vi "PostStop - Triaxial Shear (SubVI).vi"(8 "error in (no error)":errorcluster, 11 "Cluster in in":T1 {"M Event" items=["Stop", "Running", "PID", "Up Limit", "Down Limit", "Load Limit"]; "Test Type" items=["Please Select", "Triaxial Shear", "Triaxial UU", "Shearbox", "Permeability", "Consolidation (Stepped Loading)/Swelling", "Saturation (Incremental)", "User Defined", "UCT", "Isotropic Consolidation", "Swelling Pressure"]; "Data"."Test Type" items=["Please Select", "Triaxial Shear", "Triaxial UU", "Shearbox", "Permeability", "Consolidation (Stepped Loading)/Swelling", "Saturation (Incremental)", "User Defined", "UCT", "Isotropic Consolidation", "Swelling Pressure"]}) -> (0 "error out":errorcluster, 2 "Enum":T10, 3 "Cluster out":T1 {"M Event" items=["Stop", "Running", "PID", "Up Limit", "Down Limit", "Load Limit"]; "Test Type" items=["Please Select", "Triaxial Shear", "Triaxial UU", "Shearbox", "Permeability", "Consolidation (Stepped Loading)/Swelling", "Saturation (Incremental)", "User Defined", "UCT", "Isotropic Consolidation", "Swelling Pressure"]; "Data"."Test Type" items=["Please Select", "Triaxial Shear", "Triaxial UU", "Shearbox", "Permeability", "Consolidation (Stepped Loading)/Swelling", "Saturation (Incremental)", "User Defined", "UCT", "Isotropic Consolidation", "Swelling Pressure"]})   [LabVIEW 2019]
uses:
  Controls/RunTest - State.ctl
  Controls/RunTest - Data Structure.ctl
  Controls/Test Panel - Data Structure.ctl
  Controls/Station - Test Type.ctl
  <vilib>/Utility/miscctls.llb/LVRowAndColumnTypeDef.ctl
  Controls/RunTest - Calculate Data.ctl
  <vilib>/httpClient/ClientHandle.ctl
  Controls/RunTest - Start Condition.ctl
  Controls/RunTest - Stop Condition.ctl
  Controls/UDP - Event.ctl
  Controls/UDP - Command.ctl
  <vilib>/httpClient/LabVIEWHTTPClient.lvlib
panel:
  out "BP LastValue":sgl
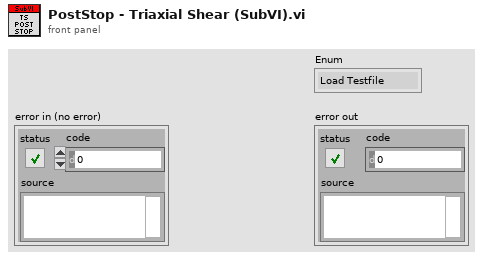
[diagram p1: front panel]
types:
  T1 = typedef "RunTest - Data Structure.ctl" = cluster{"Test Plan":string[], "PlanRow":i32, "Device Name":string[], "Timeout":i32, "Start?":bool, "Pause?":bool, "IP Address":string[], "LogRow":i32, "Logtype":u16, "Log Elapse":sgl, "Data":T2, "Stop log?":bool, "tdms":refnum<k34>, "Sensor Data":sgl[], "Start time":timestamp, "Prev Log Elapse":u32, "Plot":u16, "X-Axis":u16[], "Y-Axis":u16[], "XY":cluster{"X":dbl, "Y":dbl}[][], "End Stage?":bool, "1run":bool, "Condition":u16[], "Start Con":bool, "Log Con":bool, "Stop Con":bool, "Start Elapse":dbl, "Start Load":dbl, "Motor":i32, "StartRow":i32, "number log":i32, "Dir":bool, "Start time test":timestamp, "Auto":bool, "Check return?":bool, "Inv":cluster{"M":i32[], "Bool":bool[]}, "tdms temp":refnum<k34>, "Zero?":bool, "Plot Timer":dbl, "1st Run":bool, "TDMS Path":path, "MaxLoad":dbl, "Log Timer":sgl[], "Test Type":T3, "Log Sensor":string[], "Save?":bool, "1st Log":bool, "Y-Axis 2":u16[], "On Y-Axis 2":bool, "Decimal":u8[], "Init":cluster{"PWP TS":sgl, "Load TS":sgl, "Volume TS":sgl, "Disp TS":sgl, "CP":sgl, "Vol In":sgl, "Vol Out":sgl, "Load UCT":sgl, "Disp UCT":sgl, "PWP Sat":sgl, "CP Sat":sgl, "Volume IsoCons":sgl, "PWP IsoCons":sgl, "PWP TUU":sgl, "Load TUU":sgl, "Volume TUU":sgl, "Disp TUU":sgl, "Load Cons":sgl, "Disp Cons":sgl, "Volume Sat":sgl, "Vertical Load SB":sgl, "Vertical Disp SB":sgl, "H Disp SB":sgl, "H Load SB":sgl}, "Calc":T5, "Device Index":i32[], "Channel Index":i32[], "http ref":T6, "fileid":string, "Step Cons":cluster{"V Stress":sgl, "H Settlement":sgl}, "RunTest":bool, "Graph Last":i32, "Init?":bool, "Datalog":bool[], "Start":T7, "Stop":T8, "Running?":bool, "StartTime":dbl, "Log Prev Time":dbl, "KeyName":string[], "Test RunTime":dbl, "Log Prev Axial":dbl, "M Event":T9[], "Last Log":bool, "popup":bool, "PreStart UU":bool, "PreStart Sat":bool}
  T2 = typedef "Test Panel - Data Structure.ctl" = cluster{"Station":string, "Sample ID":string, "Job No":string, "Job Description":string, "Filename":string, "Test Type":T3, "Speciment No":string, "Depth":string, "Height":string, "Diameter/Length":string, "Weight":string, "Test Parameter":string, "Station[]":string[], "Edit Pos":T4, "Edit Pos Prev":T4, "Area":string, "Path":string}
  T3 = typedef "Station - Test Type.ctl" = u16
  T4 = typedef "LVRowAndColumnTypeDef.ctl" = cluster{"Row":i32, "Column":i32}
  T5 = typedef "RunTest - Calculate Data.ctl" = cluster{"TS":cluster{"Change PWP":sgl, "Change Vol":sgl, "Axial Load":sgl, "CiL":sgl, "Deviator":sgl, "Axial Strain":sgl, "MaxDeviator":sgl}, "TUU":cluster{"Change PWP":sgl, "Axial Load":sgl, "CiL":sgl, "Deviator":sgl, "Axial Strain":sgl, "MaxDeviator":sgl}, "Sat":cluster{"B Value":sgl, "PWP Diss":sgl, "CPP":sgl, "CV":sgl}, "Per":cluster{"Change Vol In":sgl, "Change Vol Out":sgl, "Mean Vol":sgl, "Gradient Pressure":sgl, "Outlet Flow":sgl, "Inlet Flow":sgl, "I X1":sgl, "I X2":sgl, "I Y1":sgl, "I Y2":sgl, "O X1":sgl, "O X2":sgl, "O Y1":sgl, "O Y2":sgl}, "Step Cons":cluster{"V Stress":sgl, "H Settlement":sgl, "Total H Settle":sgl, "Prev Total H":sgl}, "UCT":cluster{"ALC":sgl, "H Change":sgl, "Deviator":sgl, "Axial Strain":sgl, "V Stress":sgl, "MaxDeviator":sgl}, "ISO Cons":cluster{"CPP":sgl, "PWP Diss":sgl, "CV":sgl}, "SB":cluster{"Speci LenC":sgl, "Shear Strain":sgl, "H LC":sgl, "Normal Stress":sgl, "Shear Stress":sgl, "MaxShear":sgl}}
  T6 = typedef "LabVIEWHTTPClient.lvlib/ClientHandle.ctl" = refnum<k1>
  T7 = typedef "RunTest - Start Condition.ctl" = cluster{"Cons":cluster{"VS":dbl, "Delay":bool, "No Delay":dbl}, "Sat":cluster{"CP":dbl, "BP":dbl, "StartBP":bool, "Target CP":bool, "Target BP":bool}, "Iso":cluster{"Select":dbl, "BP":dbl, "IC2":dbl, "IC3":dbl, "IC4":dbl, ". IC6":bool, "IC6":dbl, "IC6-2":dbl, "Target":bool, "Time Cond":dbl, "Last PWP":dbl}, "TS":cluster{"SS":dbl, "Engage":bool, "ES":dbl, "LC":dbl, "PreStart":bool, "Trig SS":bool, "Drain":dbl}, "TUU":cluster{"SS":dbl, "Engage":bool, "ES":dbl, "LC":dbl, "PreStart":bool, "Trig SS":bool, "CP":dbl, "Delay Value":dbl, "Delay":bool, "CP PID":bool}, "UCT":cluster{"SS":dbl, "Engage":bool, "ES":dbl, "LC":dbl, "PreStart":bool, "Trig SS":bool}, "Enable?":bool, "SB":cluster{"SS":dbl, "Engage":bool, "ES":dbl, "LC":dbl, "PreStart":bool, "Trig SS":bool, "VS":dbl, "Delay Value":dbl, "Delay":bool, "VS PID":bool}, "Perm":cluster{"DP":dbl}}
  T8 = typedef "RunTest - Stop Condition.ctl" = cluster{"Cons":cluster{"Select":i32, "Disp":dbl, "Time":dbl, "Time2":dbl, "Disp 2":dbl, "Time Cond":dbl, "Last Disp":dbl, "Swell":bool}, "Sat":cluster{"Select":i32, "PP":dbl, "Time":dbl, "VC":dbl, "Time2":dbl, "Time Cond":dbl, "Last PP":dbl, ".B":bool, "B":dbl, "Last Vc":dbl, "Time Cond 2":dbl, "Time3":dbl, "Time Cond 3":dbl, "B Achieve":bool}, "Iso":cluster{"PP":dbl, "Time":dbl, "VC":dbl, "Time2":dbl, "Time Cond":dbl, "Last Vc":dbl, ".PP":bool, "Time Cond 2":dbl, "Select":i32}, "TS":cluster{"Axial":dbl, ".MaxDev":bool, "MaxDev Value":dbl, "Return":bool, "Reset":bool, "Prev Time":dbl, "PostStop Run":bool, "CP Stop":bool, "BP Stop":bool, "PostStop Trig":bool, "Reset Value":dbl, "BPTrig":bool, "CPTrig":bool, "VLCTrig":bool}, "TUU":cluster{"Axial":dbl, ".MaxDev":bool, "MaxDev Value":dbl, "Return":bool, "Reset":bool, "Prev Time":dbl, "PostStop Run":bool, "CP Stop":bool, "BP Stop":bool, "PostStop Trig":bool, "Reset Value":dbl, "BPTrig":bool, "CPTrig":bool, "VLCTrig":bool}, "UCT":cluster{"Axial":dbl, ".MaxDev":bool, "MaxDev Value":dbl, "Return":bool, "Reset":bool, "Prev Time":dbl, "PostStop Run":bool, "CP Stop":bool, "BP Stop":bool, "PostStop Trig":bool}, "Enable?":bool, "SB":cluster{"Shear":dbl, ".MaxShear":bool, "MaxShear Value":dbl, "Return":bool, "Reset":bool, "Prev Time":dbl, "PostStop Run":bool, "CP Stop":bool, "BP Stop":bool, "PostStop Trig":bool, "Reset Value":dbl, "BPTrig":bool, "CPTrig":bool, "VLCTrig":bool}, "Perm":cluster{"Max Time":bool, "Reset":bool, "PostStop Run":bool, "Ratio":bool, "Reset Value":dbl, "Time":dbl, "RatioTime":dbl, "RatioMore":dbl, "RatioLess":dbl, "Time Cond":dbl, "Time Cond 2":dbl, "Prev IF":dbl, "Prev OF":dbl, "PostStop Trig":bool, "BP Trig":bool, "DP Stop":bool, "BP Stop":bool, "CP Stop":bool, "CP Trig":bool}, "SP":cluster{".Max Time":bool, ".Time":bool, "Time":dbl, "MaxTime":dbl, "Time Cond":dbl, "Max Time Cond":dbl, "Stress":dbl}}
  T9 = typedef "UDP - Event.ctl" = u16
  T10 = typedef "RunTest - State.ctl" = enum16{"Load Testfile", "Notifier", "Init", "Idle", "Load", "Read DB", "Run", "Pause", "Stop", "Check Start", "Check Stop", "Check Post Stop", "Check Log", "EndStage", "Data View", "Display", "Graph", "Graph Old", "Close", "Stop PID", "Check Limit", "Auto", "Up", "Log", "Zero", "Machine Control", "Save Report"}
  T11 = typedef "UDP - Command.ctl" = enum16{"Stop", "Jog Up", "Jog Down", "Ramp Up", "Ramp Down", "PID Target", "PID Ramp", "Disp Run", "Read Ch Data", "Zero Channel", "Zero Disp", "Read Sensor", "Write Sensor", "Read ADC", "Write ADC", "Read PID", "Write PID", "Read Test", "Write Test", "Read System", "Write System", "Read Datalog", "Read Datalog Sensor"}
  T12 = cluster{"Target Load":sgl, "Target Disp":sgl, "Rate":sgl, "Speed":sgl}
  T13 = enum16{"None", "Run Target", "Run Ramp", "Run Disp"}
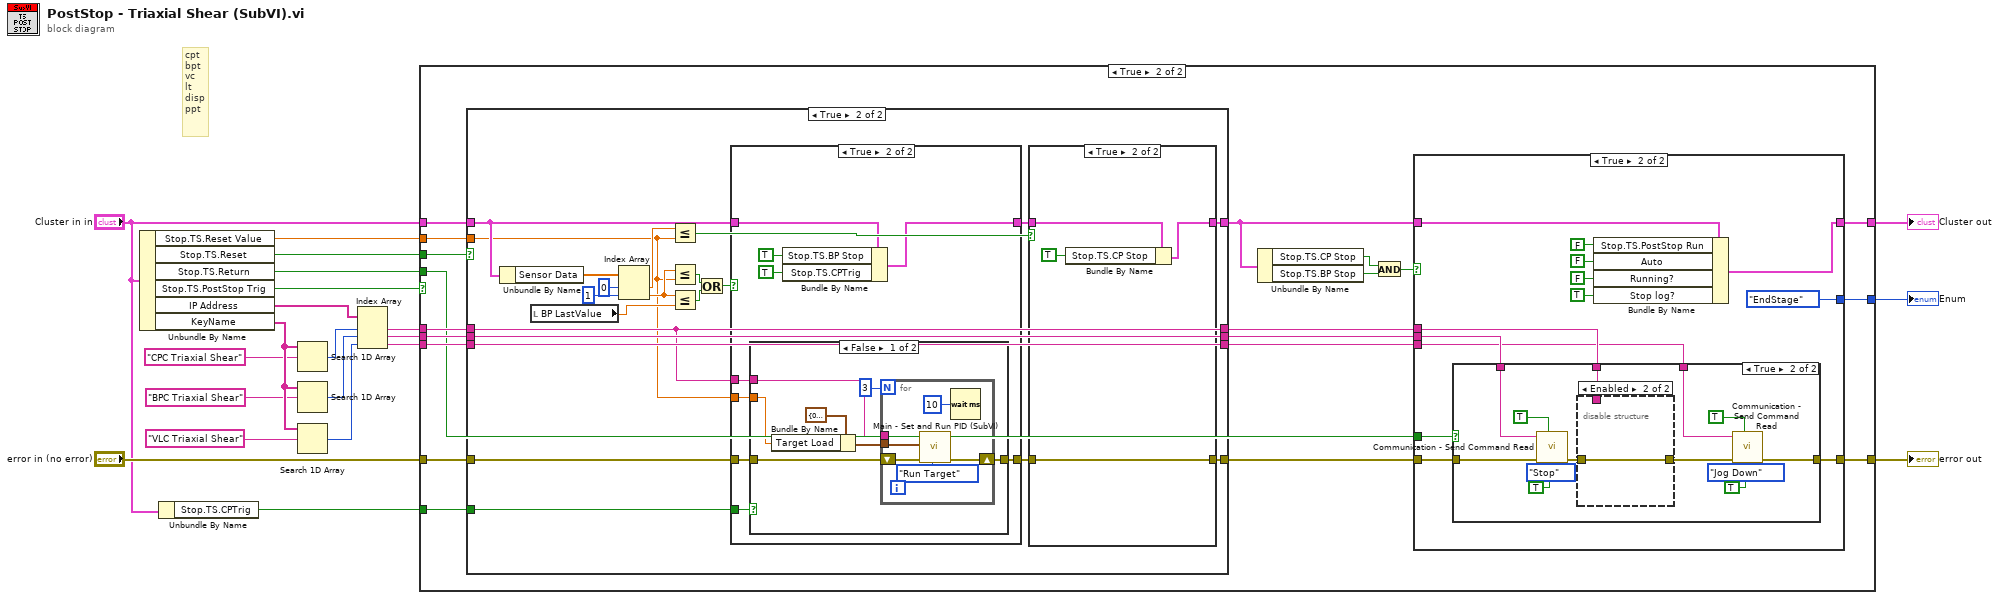
[diagram p0: block diagram]
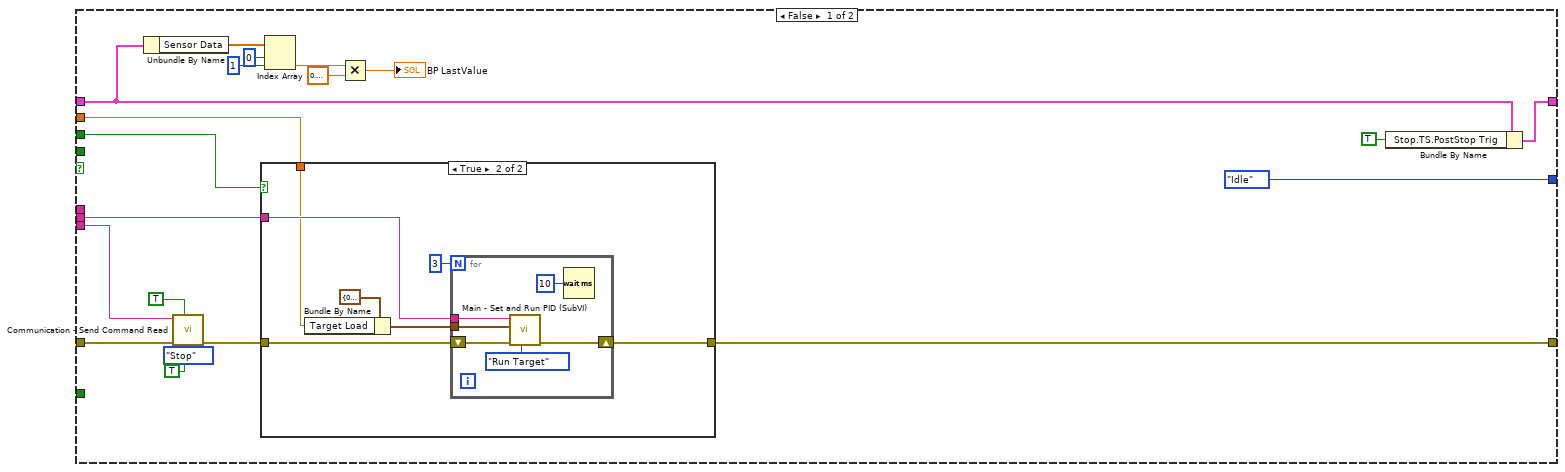
[diagram p2: hidden frame]
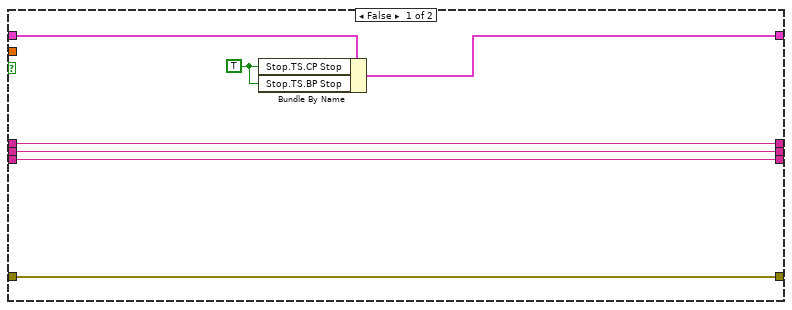
[diagram p4: hidden frame]
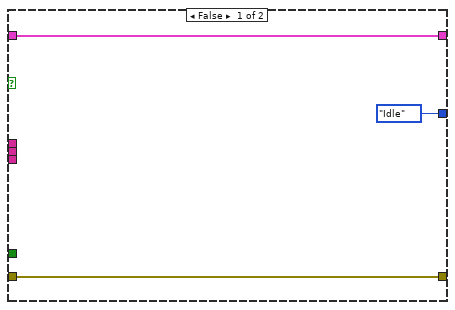
[diagram p8: hidden frame]
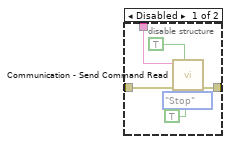
[diagram p10: hidden frame]
diagram:
  # "cpt\nbpt\nvc\nlt\ndisp\nppt"
  n1 = Unbundle By Name("Cluster in in") -> ("Stop.TS.Reset Value"=w21:dbl, "Stop.TS.Reset"=w19:bool, "Stop.TS.Return"=w18:bool, "Stop.TS.PostStop Trig"=w3:bool, "IP Address"=w20:string[], "KeyName"=w16:string[])
  n2 = Unbundle By Name("Cluster in in") -> ("Stop.TS.CPTrig"=w1:bool)
  n3 = Search 1D Array(1D array=w16, element="CPC Triaxial Shear" ("String")) -> (index of element=w9:i32)  [unwired: 1 in]
  n4 = Search 1D Array(1D array=w16, element="BPC Triaxial Shear" ("String")) -> (index of element=w10:i32)  [unwired: 1 in]
  n5 = Search 1D Array(1D array=w16, element="VLC Triaxial Shear" ("String")) -> (index of element=w15:i32)  [unwired: 1 in]
  n6 = Index Array(array=w20, index #1=w9, index #2=w10, index #3=w15) -> (element #1=w11:string, element #2=w12:string, element #3=w17:string)
  n7 = case shown="True" w3 {
    tunnel: [w41 w69] -> w4
    tunnel: "Cluster in in" -> [w25 w71]
    tunnel: [w32 w67] -> w6
    tunnel: "error in (no error)" -> [w35 w75]
    tunnel: w11 -> [_ w74]
    tunnel: w12 -> [w31 w73]
    tunnel: [RunTest_-_State."Idle" w72] -> w13
    tunnel: w17 -> [w34 w59]
    tunnel: w18 -> [_ w57]
    tunnel: w19 -> [w39 w56]
    tunnel: w21 -> [w30 w63]
    tunnel: w1 -> [_ w62]
    frame False {
      n8 = Unbundle By Name(w25) -> ("Sensor Data"=w28:sgl[])
      n9 = call "Communication - Send Command Read.vi"("Fron?"=TRUE, "Bypass?"=TRUE, "error in (no error)"=w35, "Action"=UDP_-_Command."Stop", "Device IP Address"=w34) -> ("error out"=w33:errorcluster)  [unwired: 6 in]
      n10 = case shown="True" w39 {
        tunnel: w33 -> [w42 w47]
        tunnel: w31 -> [_ w46]
        tunnel: [w42 w44] -> w32
        tunnel: w30 -> [_ w45]
        frame False {
        }
        frame True {
          n11 = Bundle By Name(cluster=T12 {"Target Load"=0.0, "Target Disp"=0.0, "Rate"=0.0, "Speed"=0.0} ("Test"), "Target Load"=w45) -> (w48:T12)
          n12 = for {
            N: 3 -> [_]
            tunnel: w48 -> [w54]
            tunnel: w46 -> [w52]
            shift-right: [w51] -> w44
            shift-left: w47 -> [w53]
            n13 = call "Main - Set and Run PID (SubVI).vi"("Action"=T13."Run Target", "error in (no error)"=w53, "Test"=w54, "IP Address"=w52) -> ("error out"=w51:errorcluster)  [unwired: 7 in]
            n14 = Wait (ms)(milliseconds to wait=u32 10) -> ()  [unwired: 1 out]
          }
        }
      }
      n15 = Index Array(array=w28, index #1=0 ("index"), index #2=1 ("index")) -> (element #2=w24:sgl)  [unwired: 1 out]
      n16 = Multiply(x=w24, y=sgl 0.3) -> (x*y=→"BP LastValue":sgl)
      n17 = Bundle By Name(cluster=w25, "Stop.TS.PostStop Trig"=TRUE) -> (w41:T1)
    }
    frame True {
      n18 = case shown="True" w56 {
        tunnel: w75 -> [w79 w103]
        tunnel: w74 -> [w78 w89]
        tunnel: w73 -> [w77 w91]
        tunnel: w71 -> [w81 w102]
        tunnel: [w80 w101] -> w68
        tunnel: [w79 w100] -> w66
        tunnel: w63 -> [_ w86]
        tunnel: w62 -> [_ w92]
        tunnel: [w78 w89] -> w61
        tunnel: [w77 w91] -> w60
        tunnel: w59 -> [w76 w90]
        tunnel: [w76 w90] -> w58
        frame False {
          w82 = TRUE ("Stop.TS.CP Stop")
          n19 = Bundle By Name(cluster=w81, "Stop.TS.CP Stop"=w82, "Stop.TS.BP Stop"=w82) -> (w80:T1)
        }
        frame True {
          n20 = Unbundle By Name(w102) -> ("Sensor Data"=w99:sgl[])
          n21 = local read "BP LastValue"() -> (w88:sgl)
          n22 = Index Array(array=w99, index #1=0 ("index"), index #2=1 ("index")) -> (element #1=w94:sgl, element #2=w87:sgl)
          n23 = Less Or Equal?(x=w94, y=w86) -> (x <= y?=w93:bool)
          n24 = Less Or Equal?(x=w87, y=w86) -> (x <= y?=w85:bool)
          n25 = Less Or Equal?(x=w87, y=w88) -> (x <= y?=w84:bool)
          n26 = Or(x=w85, y=w84) -> (x .or. y?=w83:bool)
          n27 = case shown="True" w83 {
            tunnel: w103 -> [w111 w113]
            tunnel: [w111 w117] -> w96
            tunnel: w102 -> [w110 w120]
            tunnel: [w110 w118] -> w95
            tunnel: w89 -> [_ w116]
            tunnel: w86 -> [_ w115]
            tunnel: w92 -> [_ w114]
            frame False {
            }
            frame True {
              n28 = case shown="False" w114 {
                tunnel: w113 -> [w125 w134]
                tunnel: [w124 w134] -> w117
                tunnel: w116 -> [w123 _]
                tunnel: w115 -> [w122 _]
                frame False {
                  n29 = Bundle By Name(cluster=T12 {"Target Load"=0.0, "Target Disp"=0.0, "Rate"=0.0, "Speed"=0.0} ("Test"), "Target Load"=w122) -> (w127:T12)
                  n30 = for {
                    N: 3 -> [_]
                    tunnel: w127 -> [w133]
                    tunnel: w123 -> [w129]
                    shift-right: [w130] -> w124
                    shift-left: w125 -> [w131]
                    n31 = call "Main - Set and Run PID (SubVI).vi"("Action"=T13."Run Target", "error in (no error)"=w131, "Test"=w133, "IP Address"=w129) -> ("error out"=w130:errorcluster)  [unwired: 7 in]
                    n32 = Wait (ms)(milliseconds to wait=u32 10) -> ()  [unwired: 1 out]
                  }
                }
                frame True {
                }
              }
              n33 = Bundle By Name(cluster=w120, "Stop.TS.BP Stop"=TRUE, "Stop.TS.CPTrig"=TRUE) -> (w118:T1)
            }
          }
          n34 = case shown="True" w93 {
            tunnel: w96 -> [w105 w106]
            tunnel: [w105 w106] -> w100
            tunnel: w95 -> [w104 w108]
            tunnel: [w104 w107] -> w101
            frame False {
            }
            frame True {
              n35 = Bundle By Name(cluster=w108, "Stop.TS.CP Stop"=TRUE ("Stop.TS.BP Stop")) -> (w107:T1)
            }
          }
        }
      }
      n36 = Unbundle By Name(w68) -> ("Stop.TS.CP Stop"=w65:bool, "Stop.TS.BP Stop"=w64:bool)
      n37 = And(x=w65, y=w64) -> (x .and. y?=w70:bool)
      n38 = case shown="True" w70 {
        tunnel: [RunTest_-_State."Idle" RunTest_-_State."EndStage"] -> w72
        tunnel: [w136 w147] -> w69
        tunnel: w68 -> [w136 w149]
        tunnel: [w135 w141] -> w67
        tunnel: w66 -> [w135 w144]
        tunnel: w61 -> [_ w143]
        tunnel: w60 -> [_ w142]
        tunnel: w58 -> [_ w140]
        tunnel: w57 -> [_ w139]
        frame False {
        }
        frame True {
          n39 = case shown="True" w139 {
            tunnel: w144 -> [w151 w160]
            tunnel: w143 -> [_ w159]
            tunnel: w142 -> [_ w158]
            tunnel: [w151 w153] -> w141
            tunnel: w140 -> [_ w152]
            frame False {
            }
            frame True {
              n40 = call "Communication - Send Command Read.vi"("Fron?"=TRUE, "Bypass?"=TRUE, "error in (no error)"=w160, "Action"=UDP_-_Command."Stop", "Device IP Address"=w158) -> ("error out"=w161:errorcluster)  [unwired: 6 in]
              n41 = disable-structure shown="Enabled" {
                disable-tunnel: w161 -> [w167 w171]
                disable-tunnel: w159 -> [w166 _]
                disable-tunnel: [w165 w171] -> w154
                frame Disabled {
                  n42 = call "Communication - Send Command Read.vi"("Fron?"=TRUE, "Bypass?"=TRUE, "error in (no error)"=w167, "Action"=UDP_-_Command."Stop", "Device IP Address"=w166) -> ("error out"=w165:errorcluster)  [unwired: 6 in]
                }
                frame Enabled {
                }
              }
              n43 = call "Communication - Send Command Read.vi"("Fron?"=TRUE, "Bypass?"=TRUE, "error in (no error)"=w154, "Action"=UDP_-_Command."Jog Down", "Device IP Address"=w152) -> ("error out"=w153:errorcluster)  [unwired: 6 in]
            }
          }
          n44 = Bundle By Name(cluster=w149, "Stop.TS.PostStop Run"=FALSE, "Auto"=FALSE, "Running?"=FALSE, "Stop log?"=TRUE) -> (w147:T1)
        }
      }
    }
  }
  "Enum" <- w13
  "error out" <- w6
  "Cluster out" <- w4
